vi "init.vi"(8 "error in (no error)":errorcluster, 11 "Protocol_Generic in":refnum<class "Protocol_Generic.lvclass">) -> (0 "error out":errorcluster, 3 "Protocol_Generic out":refnum<class "Protocol_Generic.lvclass">)   [LabVIEW 2011, in "Protocol_Generic.lvclass"]
uses:
  Protocol_Generic.lvclass
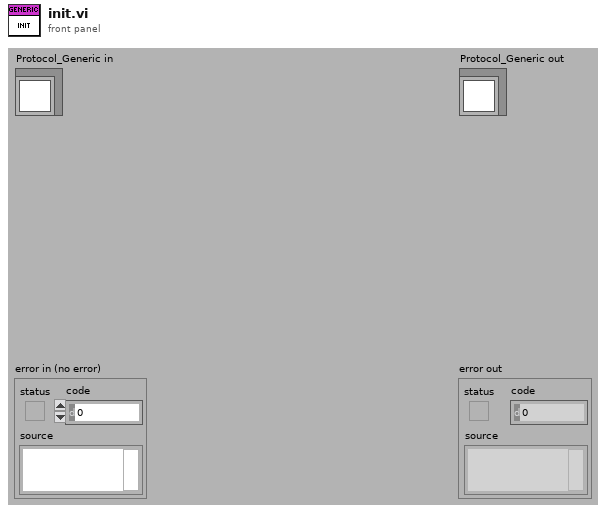
[diagram p1: front panel]
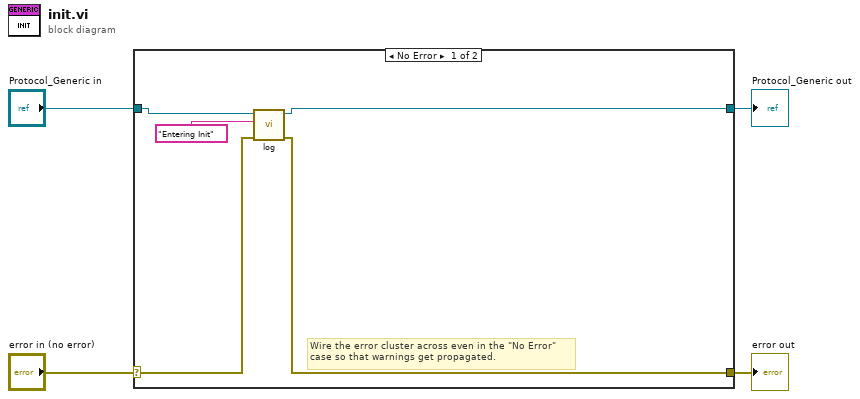
[diagram p0: block diagram]
diagram:
  n1 = case shown="No Error" "error in (no error)" {
    selector: "error in (no error)" -> [w8 w11]
    tunnel: [w7 w11] -> w3
    tunnel: [w5 w10] -> w1
    tunnel: "Protocol_Generic in" -> [w9 w10]
    frame No Error {
      # "Wire the error cluster across even in the \"No Error\"\ncase so that warnings get propagated."
      n2 = call-dynamic "log.vi"("error in (no error)"=w8, "logLineIn"="Entering Init", "Protocol_Generic in"=w9) -> ("error out"=w7:errorcluster, "Protocol_Generic out"=w5:refnum<class "Protocol_Generic.lvclass">)  [unwired: 7 in]
    }
    frame Error {
    }
  }
  "error out" <- w3
  "Protocol_Generic out" <- w1
